vi "Deadzone.vi"(2 "DeadZone":dbl, 3 "In":dbl) -> (0 "Activated":bool, 1 "Out":dbl)   [LabVIEW 2018]
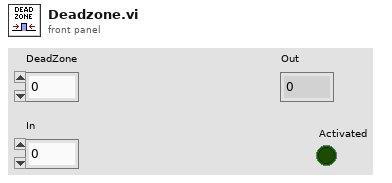
[diagram p1: front panel]
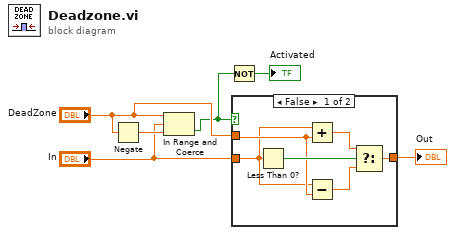
[diagram p0: block diagram]
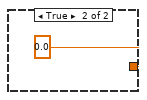
[diagram p2: hidden frame]
diagram:
  n1 = Negate(x="DeadZone") -> (-x=w6:dbl)
  n2 = In Range and Coerce(upper limit="DeadZone", x="In", lower limit=w6) -> (In Range?=w2:bool)  [unwired: 1 out]
  n3 = Not(x=w2) -> (.not. x?=→"Activated":bool)
  n4 = case shown="False" w2 {
    tunnel: [w7 0.0 ("t")] -> w5
    tunnel: "In" -> [w10 _]
    tunnel: "DeadZone" -> [w11 _]
    frame False {
      n5 = Less Than 0?(x=w10) -> (x < 0?=w12:bool)
      n6 = Add(x=w10, y=w11) -> (x+y=w8:dbl)
      n7 = Subtract(x=w10, y=w11) -> (x-y=w9:dbl)
      n8 = Select(t=w8, s=w12, f=w9) -> (s? t:f=w7:dbl)
    }
    frame True {
    }
  }
  "Out" <- w5
